vi "Integrate_16.vi"(11 "New samples in":u64) -> (0 "Next Sample":u8, 3 "Sum out":u16)   [LabVIEW 2014]
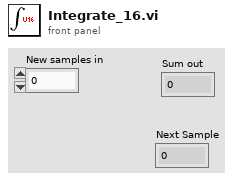
[diagram p1: front panel]
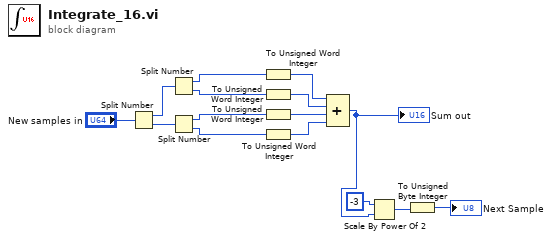
[diagram p0: block diagram]
diagram:
  n1 = Split Number(x="New samples in") -> (hi(x)=w14:u32, lo(x)=w13:u32)
  n2 = Split Number(x=w14) -> (hi(x)=w4:u16, lo(x)=w3:u16)
  n3 = Split Number(x=w13) -> (hi(x)=w2:u16, lo(x)=w1:u16)
  n4 = To Unsigned Word Integer(number=w4) -> (unsigned 16bit integer=w12:u16)
  n5 = To Unsigned Word Integer(number=w3) -> (unsigned 16bit integer=w11:u16)
  n6 = To Unsigned Word Integer(number=w2) -> (unsigned 16bit integer=w10:u16)
  n7 = To Unsigned Word Integer(number=w1) -> (unsigned 16bit integer=w9:u16)
  n8 = Compound Arithmetic op=ADD(w12, w11, w10, w9) -> (w7:u16)
  "Sum out" <- w7
  n9 = Scale By Power Of 2(n=i16 -3, x=w7) -> (x*2^n=w6:u16)
  n10 = To Unsigned Byte Integer(number=w6) -> (unsigned 8bit integer=→"Next Sample":u8)
